vi "Teleop.vi"(10 "Match Info":T1={"Autonomous Elapsed Seconds"=0.0, "TeleOp Elapsed Seconds"=0.0, "Disabled Elapsed Seconds"=0.0, "Visited Autonomous"=FALSE, "Visited TeleOp"=FALSE, "Visited Disabled"=FALSE, "Autonomous Settings"={"Autonomous Style"=enum."Independent", "VI Refnum"=refnum}}, 11 "Call Context":T2) -> ()   [LabVIEW 2014]
doc: "This VI is called for each TeleOp packet received from the DS where the robot is not disabled. It is often used to read from the joysticks and update I/O or to update setpoints for timed control loops. It should complete and return within 20 milliseconds or it may miss DS packets."
uses:
  <vilib>/Rock Robotics/WPI/DriverStation/WPI_DriverStationDerivedRobotMode.ctl
  <vilib>/Rock Robotics/WPI/DriverStation/WPI_DriverStationMatch Info.ctl
  <vilib>/Rock Robotics/WPI/RobotDrive/WPI_RobotDriveGetSetRefNum.vi
  <vilib>/Rock Robotics/WPI/Joystick/WPI_JoystickGetSetRefNum.vi
  Robot Global Data.vi
  <vilib>/Rock Robotics/Network Tables/SD Write Boolean Array.vi
  <vilib>/Rock Robotics/Network Tables/SD Write Numeric Array.vi
  <vilib>/Rock Robotics/Network Tables/SD Write Number.vi
  <vilib>/Rock Robotics/WPI/RobotDrive/WPI_RobotDriveMecanumDrive_Cartesian.vi
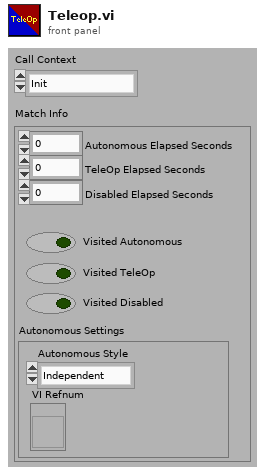
[diagram p1: front panel]
types:
  T1 = typedef "WPI_DriverStationMatch Info.ctl" = cluster{"Autonomous Elapsed Seconds":dbl, "TeleOp Elapsed Seconds":dbl, "Disabled Elapsed Seconds":dbl, "Visited Autonomous":bool, "Visited TeleOp":bool, "Visited Disabled":bool, "Autonomous Settings":cluster{"Autonomous Style":enum16{"Iterative", "Independent"}, "VI Refnum":refnum<vi>}}
  T2 = typedef "WPI_DriverStationDerivedRobotMode.ctl" = enum16{"Init", "Execute", "Stop"}
  T3 = typedef "WPI_JoystickDevRef.ctl" = cluster{"Device":T4}
  T4 = typedef "WPI_JoystickDeviceEnum.ctl" = enum16{"USB 0", "USB 1", "USB 2", "USB 3", "USB 4", "USB 5"}
  T5 = cluster{"Buttons[0]":bool, "Buttons[1]":bool, "Buttons[2]":bool, "Buttons[3]":bool, "Buttons[4]":bool, "Buttons[5]":bool, "Buttons[6]":bool, "Buttons[7]":bool, "Buttons[8]":bool}
  T6 = cluster{"Axes[0]":dbl, "Axes[1]":dbl, "Axes[2]":dbl, "Axes[3]":dbl, "Axes[4]":dbl, "Axes[5]":dbl, "Axes[6]":dbl, "Axes[7]":dbl, "Axes[8]":dbl}
  T7 = typedef "WPI_MotorControlDeviceRef.ctl" = cluster{"DeviceStatus":errorcluster, "Type":T8, "PWM":cluster{"Controller":T9, "PWM Channel":T10, "DeadBand":T11}, "CAN":cluster{"Device Number":u8, "Control Mode":T12, "Semaphore":T13, "Max Vout":dbl, "TalonSRX Control Mode":T14}, "Invert":bool, "TransformRef":T15, "InvTransformRef":T15}
  T8 = typedef "WPI_MotorControlType.ctl" = enum16{"PWM", "CAN", "CANTalonSRX"}
  T9 = typedef "FPGA_TypedefDigitalModule.ctl" = enum16{"Controller 1"}
  T10 = typedef "FPGA_DIOPWMChannel.ctl" = enum8{"PWM 0", "PWM 1", "PWM 2", "PWM 3", "PWM 4", "PWM 5", "PWM 6", "PWM 7", "PWM 8", "PWM 9", "PWM MXP 0", "PWM MXP 1", "PWM MXP 2", "PWM MXP 3", "PWM MXP 4", "PWM MXP 5", "PWM MXP 6", "PWM MXP 7", "PWM MXP 8", "PWM MXP 9", "Invalid"}
  T11 = typedef "WPI_PWMDeadband.ctl" = cluster{"Name":string, "maxPositivePwm":i32, "minPositivePwm":i32, "centerPwm":i32, "maxNegativePwm":i32, "minNegativePwm":i32, "angularRange":u16}
  T12 = typedef "WPI_CANJaguar_ControlMode.ctl" = enum8{"Percent VBus", "Current", "Speed", "Position", "Voltage"}
  T13 = typedef "Semaphore RefNum" = refnum<k1>
  T14 = typedef "WPI_CANTalonSRX_APIControlMode.ctl" = enum8{"Percent VBus", "Speed", "Position", "Slave", "Unchanged / Invalid"}
  T15 = typedef "WPI_PWMTransform_ConPane.ctl" = refnum<vi>
  T16 = typedef "WPI_ServoDeviceRef.ctl" = cluster{"DeviceStatus":errorcluster, "Controller":T9, "PWM Channel":T10, "DeadBand":T11}
  T17 = typedef "WPI_RobotDriveDevRef.ctl" = cluster{"DevStatus":errorcluster, "Motors[]":T7[], "Square Inputs":bool, "Max Output":dbl}
  T18 = typedef "WPI_GyroDevRef.ctl" = cluster{"DevStatus":errorcluster, "Analog Module":T19, "Analog Channel":T20, "Offset":dbl, "Gain (VoltsPerDegree/Second)":dbl}
  T19 = typedef "FPGA_TypedefAnalogModule.ctl" = enum16{"Controller 1"}
  T20 = typedef "FPGA_AIChannel.ctl" = enum8{"AI 0", "AI 1", "AI 2", "AI 3", "AI MXP 0", "AI MXP 1", "AI MXP 2", "AI MXP 3", "Invalid"}
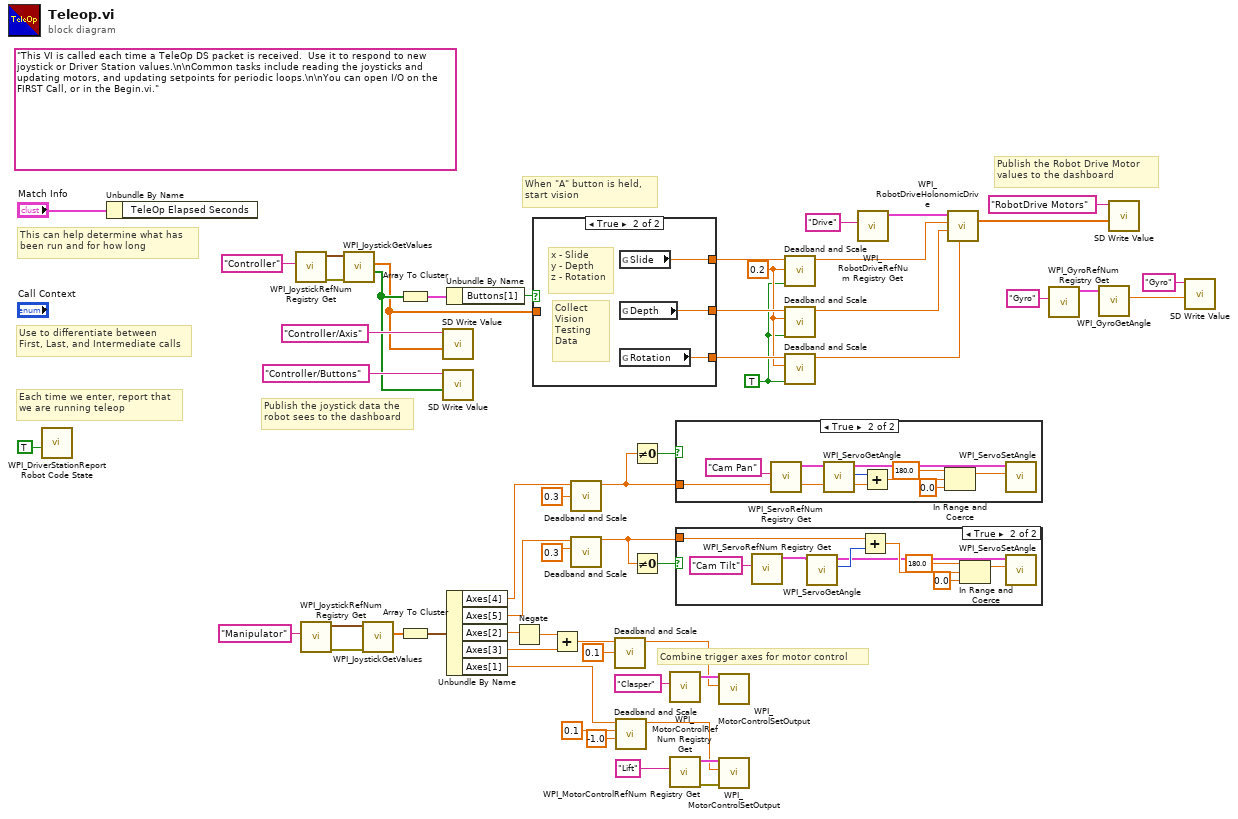
[diagram p0: block diagram]
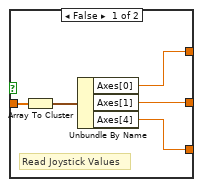
[diagram p4: hidden frame]
diagram:
  w29 = TRUE
  w33 = 0.2
  (unwired) "This VI is called each time a TeleOp DS packet is received.  Use it to respond to new joystick or Driver Station values.\n\nCommon tasks include reading the joysticks and updating motors, and updating setpoints for periodic loops.\n\nYou can open I/O on the FIRST Call, or in the Begin.vi."
  # "Combine trigger axes for motor control"
  # "When \"A\" button is held,\nstart vision"
  # "Publish the Robot Drive Motor\nvalues to the dashboard"
  # "Publish the joystick data the\nrobot sees to the dashboard"
  # "Each time we enter, report that\nwe are running teleop"
  # "Use to differentiate between\nFirst, Last, and Intermediate calls"
  # "This can help determine what has\nbeen run and for how long"
  n1 = call <vilib>:"WPI_DriverStationReport Robot Code State.vi"("TeleOp"=TRUE ("Autonomous")) -> ()  [unwired: 10 in, 1 out]
  n2 = Unbundle By Name("Match Info") -> ()  [unwired: 1 out]
  n3 = call <vilib>:"WPI_JoystickRefNum Registry Get.vi"("refnum name"="Controller") -> ("error out"=w45:errorcluster, "JoystickDevRef"=w46:T3)  [unwired: 1 in, 8 out]
  n4 = call <vilib>:"WPI_JoystickRefNum Registry Get.vi"("refnum name"="Manipulator") -> ("error out"=w25:errorcluster, "JoystickDevRef"=w21:T3)  [unwired: 9 in]
  n5 = call <vilib>:"WPI_JoystickGetValues.vi"("error in (no error)"=w45, "JoystickDevRef"=w46) -> ("Buttons"=w44:bool[], "Axes"=w37:dbl[])  [unwired: 5 in, 3 out]
  n6 = call <vilib>:"WPI_JoystickGetValues.vi"("error in (no error)"=w25, "JoystickDevRef"=w21) -> ("Axes"=w9:dbl[])  [unwired: 5 in, 4 out]
  n7 = Array To Cluster(array=w44) -> (cluster=w43:T5)
  n8 = Array To Cluster(array=w9) -> (cluster=w27:T6)
  n9 = call-poly <vilib>:"SD Write Value.vi"("Numeric Array"=w37, "Name"="Controller/Axis") -> ()  [unwired: 8 in, 2 out]
  n10 = call-poly <vilib>:"SD Write Value.vi"("Boolean Array"=w44, "Name"="Controller/Buttons") -> ()  [unwired: 8 in, 2 out]
  n11 = Unbundle By Name(w43) -> ("Buttons[1]"=w42:bool)
  n12 = Unbundle By Name(w27) -> ("Axes[4]"=w2:dbl, "Axes[5]"=w4:dbl, "Axes[2]"=w18:dbl, "Axes[3]"=w16:dbl, "Axes[1]"=w11:dbl)
  n13 = Negate(x=w18) -> (-x=w17:dbl)
  n14 = case shown="True" w42 {
    tunnel: [w57 w63] -> w34
    tunnel: [w58 w62] -> w35
    tunnel: [w56 w61] -> w36
    tunnel: w37 -> [w59 _]
    frame False {
      # "Read Joystick Values"
      n15 = Array To Cluster(array=w59) -> (cluster=w60:T6)
      n16 = Unbundle By Name(w60) -> ("Axes[0]"=w57:dbl, "Axes[1]"=w58:dbl, "Axes[4]"=w56:dbl)
    }
    frame True {
      # "Collect Vision Testing Data"
      # "x - Slide\ny - Depth\nz - Rotation"
      n17 = global read "Robot Global Data.vi" "Slide"() -> (w63:dbl)
      n18 = global read "Robot Global Data.vi" "Depth"() -> (w62:dbl)
      n19 = global read "Robot Global Data.vi" "Rotation"() -> (w61:dbl)
    }
  }
  n20 = Add(x=w17, y=w16) -> (x+y=w14:dbl)
  n21 = call "Deadband and Scale.vi"("Dead Zone (abs)"=0.3, "Input"=w2) -> ("Output"=w3:dbl)  [unwired: 9 in]
  n22 = call "Deadband and Scale.vi"("Dead Zone (abs)"=0.3, "Input"=w4) -> ("Output"=w6:dbl)  [unwired: 9 in]
  n23 = call "Deadband and Scale.vi"("Dead Zone (abs)"=0.1, "Input"=w14) -> ("Output"=w15:dbl)  [unwired: 9 in]
  n24 = call "Deadband and Scale.vi"("Scaler"=-1.0, "Dead Zone (abs)"=0.1, "Input"=w11) -> ("Output"=w13:dbl)  [unwired: 8 in]
  n25 = Not Equal To 0?(x=w3) -> (x != 0?=w7:bool)
  n26 = Not Equal To 0?(x=w6) -> (x != 0?=w8:bool)
  n27 = call <vilib>:"WPI_MotorControlRefNum Registry Get.vi"("refnum name"="Clasper") -> ("MotorControlDevRef"=w22:T7)  [unwired: 9 in, 1 out]
  n28 = call <vilib>:"WPI_MotorControlRefNum Registry Get.vi"("refnum name"="Lift") -> ("error out"=w20:errorcluster, "MotorControlDevRef"=w19:T7)  [unwired: 9 in]
  n29 = case shown="True" w7 {
    tunnel: w3 -> [_ w72]
    frame False {
    }
    frame True {
      n30 = call <vilib>:"WPI_ServoRefNum Registry Get.vi"("refnum name"="Cam Pan") -> ("ServoDeviceRef"=w70:T16)  [unwired: 9 in, 1 out]
      n31 = call <vilib>:"WPI_ServoGetAngle.vi"("ServoDeviceRef"=w70) -> ("ServoDeviceRef"=w64:T16, "Angle"=w69:u16)  [unwired: 7 in, 1 out]
      n32 = Add(x=w69, y=w72) -> (x+y=w68:dbl)
      n33 = In Range and Coerce(upper limit=180.0, x=w68, lower limit=0.0) -> (coerced(x)=w65:dbl)  [unwired: 1 out]
      n34 = call <vilib>:"WPI_ServoSetAngle.vi"("Angle"=w65, "ServoDeviceRef"=w64) -> ()  [unwired: 8 in, 2 out]
    }
  }
  n35 = case shown="True" w8 {
    tunnel: w6 -> [_ w81]
    frame False {
    }
    frame True {
      n36 = call <vilib>:"WPI_ServoRefNum Registry Get.vi"("refnum name"="Cam Tilt") -> ("ServoDeviceRef"=w79:T16)  [unwired: 9 in, 1 out]
      n37 = call <vilib>:"WPI_ServoGetAngle.vi"("ServoDeviceRef"=w79) -> ("ServoDeviceRef"=w73:T16, "Angle"=w78:u16)  [unwired: 7 in, 1 out]
      n38 = Add(x=w81, y=w78) -> (x+y=w77:dbl)
      n39 = In Range and Coerce(upper limit=180.0, x=w77, lower limit=0.0) -> (coerced(x)=w74:dbl)  [unwired: 1 out]
      n40 = call <vilib>:"WPI_ServoSetAngle.vi"("Angle"=w74, "ServoDeviceRef"=w73) -> ()  [unwired: 8 in, 2 out]
    }
  }
  n41 = call <vilib>:"WPI_MotorControlSetOutput.vi"("Output"=w15, "MotorControlDevRef"=w22) -> ()  [unwired: 7 in, 3 out]
  n42 = call <vilib>:"WPI_MotorControlSetOutput.vi"("error in (no error)"=w20, "Output"=w13, "MotorControlDevRef"=w19) -> ()  [unwired: 6 in, 3 out]
  n43 = call "Deadband and Scale.vi"("Square Inputs"=w29, "Dead Zone (abs)"=w33, "Input"=w34) -> ("Output"=w30:dbl)  [unwired: 8 in]
  n44 = call "Deadband and Scale.vi"("Square Inputs"=w29, "Dead Zone (abs)"=w33, "Input"=w35) -> ("Output"=w31:dbl)  [unwired: 8 in]
  n45 = call "Deadband and Scale.vi"("Square Inputs"=w29, "Dead Zone (abs)"=w33, "Input"=w36) -> ("Output"=w32:dbl)  [unwired: 8 in]
  n46 = call <vilib>:"WPI_RobotDriveRefNum Registry Get.vi"("refnum name"="Drive") -> ("RobotDriveDevRef"=w53:T17)  [unwired: 1 in, 9 out]
  n47 = call-poly <vilib>:"WPI_RobotDriveHolonomicDrive.vi"("Rotation"=w32, "Y"=w31, "X"=w30, "RobotDriveDevRef"=w53) -> ("Motor Values"=w47:dbl[])  [unwired: 5 in, 2 out]
  n48 = call <vilib>:"WPI_GyroRefNum Registry Get.vi"("refnum name"="Gyro") -> ("GyroDevRef"=w40:T18)  [unwired: 9 in, 1 out]
  n49 = call <vilib>:"WPI_GyroGetAngle.vi"("GyroDevRef"=w40) -> ("Angle"=w38:dbl)  [unwired: 7 in, 3 out]
  n50 = call-poly <vilib>:"SD Write Value.vi"("Numeric Array"=w47, "Name"="RobotDrive Motors") -> ()  [unwired: 8 in, 2 out]
  n51 = call-poly <vilib>:"SD Write Value.vi"("Numeric"=w38, "Name"="Gyro") -> ()  [unwired: 8 in, 2 out]
